vi "init.vi"(8 "error in":errorcluster, 10 "TBM module configuration in":refnum<class "TBM module configuration.lvclass">, 11 "TEC runtime in":refnum<class "TEC runtime.lvclass">) -> (0 "error out":errorcluster, 1 "data allocations":T1, 2 "execution settings":T4, 3 "TEC runtime out":refnum<class "TEC runtime.lvclass">)   [LabVIEW 2013, in "TEC runtime.lvclass"]
doc: "Provides an interface for initializing a module at runtime. While this interface performs no operations, a child should provide an override which may open any necessary references or sessions, allocate necessary memory, and perform any final configuration validataion before providing the full configuration <b>execution data</b> to the calling process."
uses:
  TEC runtime.lvclass
  <vilib>/NI/Tag Bus Module Framework/module configuration/TBM module configuration.lvclass
  <vilib>/NI/Tag Bus Module Framework/runtime/execution settings.ctl
  <vilib>/NI/Tag Bus Module Framework/channel/data tables.ctl
  <vilib>/NI/Tag Bus/dictionary/data dictionary.lvclass
  <vilib>/NI/Tag Bus/dictionary table pair.ctl
  <vilib>/NI/Tag Bus/table/data table.ctl
  configuration/TEC configuration.lvclass
  configuration/TEC configuration.lvclass/TEC configuration.ctl
  TEC runtime.lvclass/TEC runtime.ctl
  configuration/Read send to address.vi
  configuration/Read send to port.vi
  configuration/Read receive on port.vi
  configuration/Read send from port.vi
  <vilib>/NI/Tag Bus Module Framework/channel/TBM channel.lvclass
  <vilib>/NI/Tag Bus Module Framework/runtime/TBM module execution interface.lvclass
  <vilib>/NI/Tag Bus/tag bus.lvlib
  <vilib>/NI/Tag Bus/table/data table.lvlib
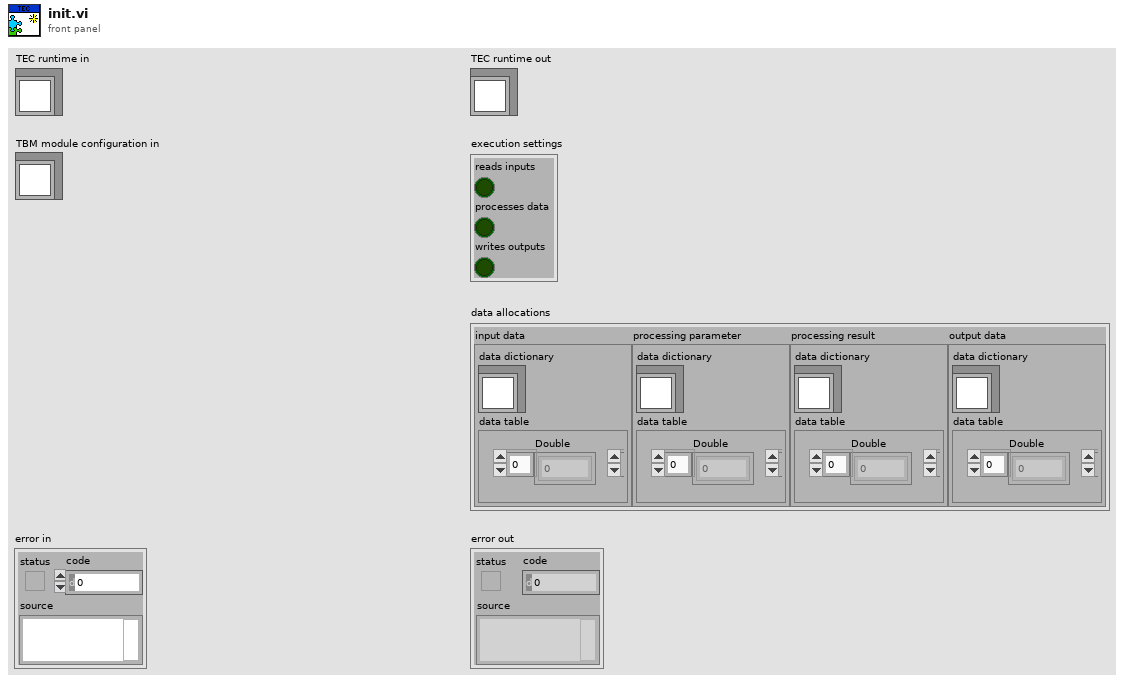
[diagram p1: front panel]
types:
  T1 = typedef "TBM channel.lvclass/data tables.ctl" = cluster{"input data":T2, "processing parameter":T2, "processing result":T2, "output data":T2}
  T2 = typedef "tag bus.lvlib/dictionary table pair.ctl" = cluster{"data dictionary":refnum<class "data dictionary.lvclass">, "data table":T3}
  T3 = typedef "tag bus.lvlib/data table.lvlib/data table.ctl" = cluster{"Double":dbl[], "Single":sgl[], "I64":i64[], "I32":i32[], "I16":i16[], "I8":i8[], "U64":u64[], "U32":u32[], "U16":u16[], "U8":u8[], "Boolean":bool[], "String":string[], "Array of Double":cluster{"DBL Array":dbl[]}[], "Array of Single":cluster{"SGL Array":sgl[]}[], "Array of I64":cluster{"I64 Array":i64[]}[], "Array of I32":cluster{"I32 Array":i32[]}[], "Array of I16":cluster{"I16 Array":i16[]}[], "Array of I8":cluster{"I8 Array":i8[]}[], "Array of U64":cluster{"U64 Array":u64[]}[], "Array of U32":cluster{"U32 Array":u32[]}[], "Array of U16":cluster{"U16 Array":u16[]}[], "Array of U8":cluster{"U8 Array":u8[]}[], "Array of Boolean":cluster{"Boolean Array":bool[]}[], "Array of String":cluster{"String Array":string[]}[]}
  T4 = typedef "TBM module execution interface.lvclass/execution settings.ctl" = cluster{"reads inputs":bool, "processes data":bool, "writes outputs":bool}
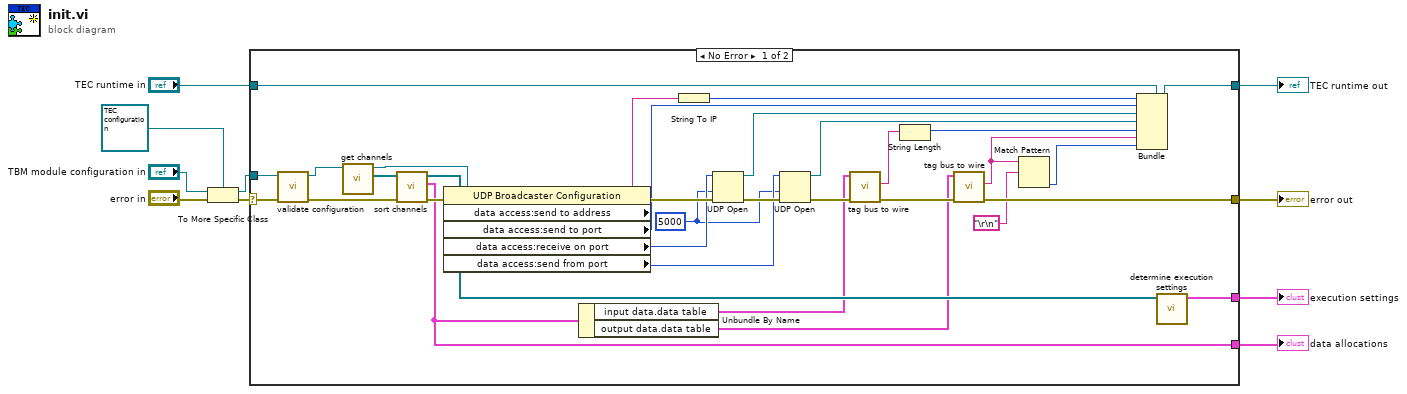
[diagram p0: block diagram]
diagram:
  n1 = To More Specific Class(target class=refnum<class "TEC configuration.lvclass"> refnum ("TEC configuration"), reference="TBM module configuration in", error in="error in") -> (specific class reference=w9:refnum<class "TEC configuration.lvclass">, error out=w10:errorcluster)
  n2 = case shown="No Error" w10 {
    selector: w10 -> [w38 w43]
    tunnel: w9 -> [w34 _]
    tunnel: "TEC runtime in" -> [w42 w44]
    tunnel: [w35 w44] -> w1
    tunnel: [w14 w43] -> w5
    tunnel: [w18 _] -> w3
    tunnel: [w41 _] -> w4
    frame No Error {
      w22 = 5000 ("timeout ms (25000)")
      n3 = call-dynamic "validate configuration.vi"("error in"=w38, "TEC configuration in"=w34) -> ("error out"=w39:errorcluster, "TEC configuration out"=w37:refnum<class "TEC configuration.lvclass">)  [unwired: 8 in]
      n4 = call-dynamic "get channels.vi"("TEC configuration in"=w37) -> ("channels"=w36:refnum<class "TBM channel.lvclass">[], "TEC configuration out"=w31:refnum<class "TEC configuration.lvclass">)  [unwired: 9 in]
      n5 = call <vilib>:"sort channels.vi"("error in"=w39, "channels in"=w36) -> ("error out"=w33:errorcluster, "data allocations"=w18:T1, "channels out"=w40:refnum<class "TBM channel.lvclass">[])  [unwired: 7 in]
      n6 = property class="UDP Broadcaster Configuration"(reference=w31, error in=w33) -> (error out=w32:errorcluster, "data access:send to address"=w28:string, "data access:send to port"=w30:u16, "data access:receive on port"=w23:u16, "data access:send from port"=w24:u16)  [unwired: 1 out]
      n7 = Unbundle By Name(w18) -> ("input data.data table"=w17:T3, "output data.data table"=w15:T3)
      n8 = String To IP(1:w28) -> (0:w29:u32)
      n9 = UDP Open(8:w32, 9:w22, 11:w23) -> (port=w25:refnum<k16>, 0:w27:errorcluster)  [unwired: 2 in, 1 out]
      n10 = UDP Open(8:w27, 9:w22, 11:w24) -> (port=w26:refnum<k16>, 0:w20:errorcluster)  [unwired: 2 in, 1 out]
      n11 = call "tag bus to wire.vi"("error in"=w20, "data table in"=w17) -> ("error out"=w16:errorcluster, "wire data"=w21:string)  [unwired: 7 in, 1 out]
      n12 = String Length(string=w21) -> (length=w19:i32)
      n13 = call "tag bus to wire.vi"("error in"=w16, "data table in"=w15) -> ("error out"=w14:errorcluster, "wire data"=w13:string)  [unwired: 7 in, 1 out]
      n14 = Match Pattern(string=w13, regular expression="\r\n") -> (offset past match=w11:i32)  [unwired: 1 in, 3 out]
      n15 = Bundle(cluster=w42, w29, w30, w25, w26, w19, w13, w11) -> (w35:refnum<class "TEC runtime.lvclass">)
      n16 = call <vilib>:"determine execution settings.vi"("channels"=w40) -> ("execution settings"=w41:T4)  [unwired: 10 in]
    }
    frame Error {
    }
  }
  "error out" <- w5
  "TEC runtime out" <- w1
  "execution settings" <- w4
  "data allocations" <- w3
